vi "Queue Nested Status.vi"(11 "Hello World Event in":refnum<class "Hello World Event.lvclass">) -> (0 "Queue Nested Count":i32, 1 "Queue Nested Aliases":string[](array[string]), 2 "Any Exist?":bool)   [LabVIEW 2021, in "Hello World Event.lvlib" / "Hello World Event.lvclass"]
uses:
  Hello World Event.lvclass
  Hello World Event.lvclass/Hello World Event.ctl
  jettl/Event jettl/Event jettl.lvclass
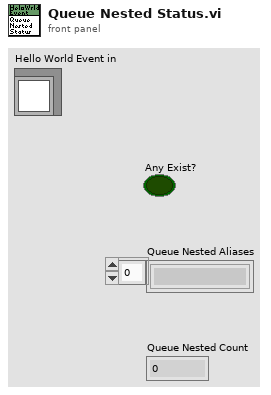
[diagram p1: front panel]
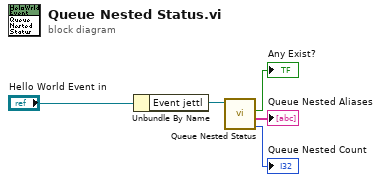
[diagram p0: block diagram]
diagram:
  n1 = Unbundle By Name("Hello World Event in") -> ("Event jettl"=w4:refnum<class "Event jettl.lvclass">)
  n2 = call-dynamic "Queue Nested Status.vi"("jettl in"=w4) -> ("Queue Nested Count"=→"Queue Nested Count":i32, "Queue Nested Aliases"=→"Queue Nested Aliases":string[], "Any Exist?"=→"Any Exist?":bool)  [unwired: 8 in]
